vi "Close.vi"(8 "error in (no error)":errorcluster, 11 "Socket Listener in":refnum<class "Socket Listener.lvclass">) -> (0 "error out":errorcluster)   [LabVIEW 2021, in "Sockets.lvlib" / "Socket Listener.lvclass"]
doc: "Closes a socket listener.\nWebSockets 2.0.1.40\nSam Sharp - MediaMongrels Ltd\nCopyright (c) 2019, MediaMongrels Ltd"
uses:
  Socket Listener.lvclass
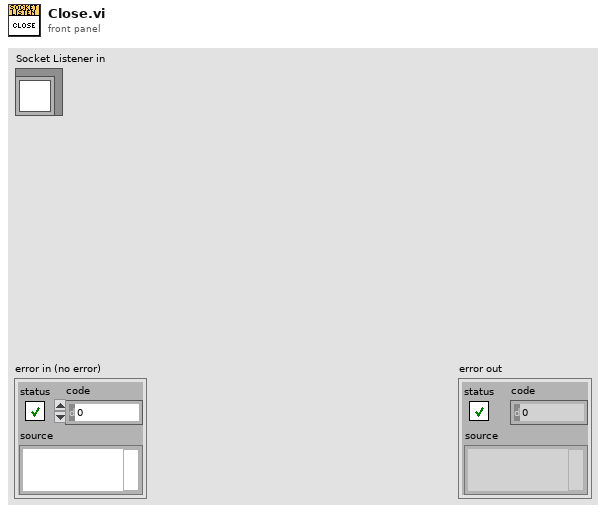
[diagram p1: front panel]
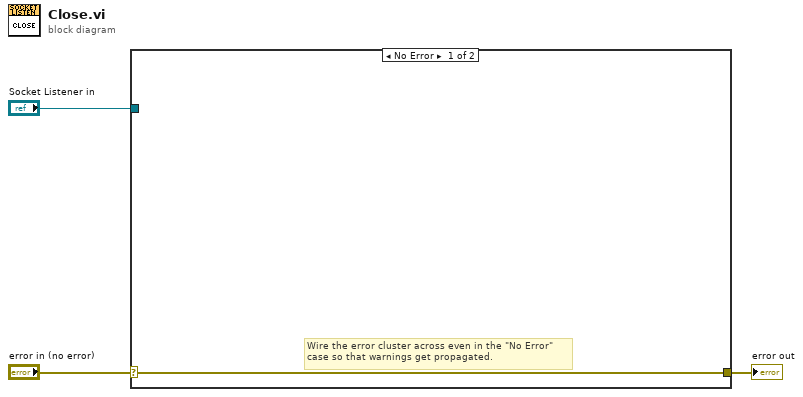
[diagram p0: block diagram]
diagram:
  n1 = case shown="No Error" "error in (no error)" {
    selector: "error in (no error)" -> [w4 w5]
    tunnel: [w4 w5] -> w2
    tunnel: "Socket Listener in" -> [_ _]
    frame No Error {
      # "Wire the error cluster across even in the \"No Error\"\ncase so that warnings get propagated."
    }
    frame Error {
    }
  }
  "error out" <- w2
